vi "NumericWeightedAverage.vi"(1 "alpha":dbl=0.6, 2 "Xcurrent":dbl(slide) scale=-5.0..5.0) -> (0 "weighted average":dbl)   [LabVIEW 2020]
panel:
  # "Xcurrent = Xcurrent * alpha + Xprevious * (1-alpha)\nmakes a weighted average"
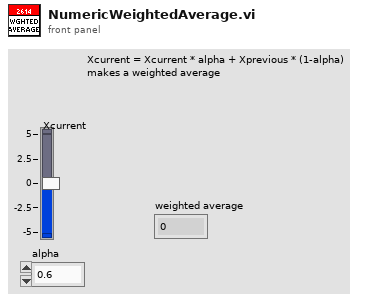
[diagram p1: front panel]
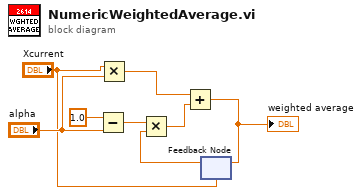
[diagram p0: block diagram]
diagram:
  n1 = Subtract(x=1.0, y="alpha") -> (x-y=w5:dbl)
  n2 = Multiply(x="Xcurrent", y="alpha") -> (x*y=w6:dbl)
  n3 = feedback #1("Xcurrent") -> (w4:dbl)
  n4 = Multiply(x=w5, y=w4) -> (x*y=w3:dbl)
  n5 = Add(x=w6, y=w3) -> (x+y=w2:dbl)
  "weighted average" <- w2
  n6 = feedback-in #1(w2) -> ()
